vi "main.vi"() -> ()   [LabVIEW 2017]
uses:
  <vilib>/Instr/_visa.llb/VISA Set IO Buffer Mask.ctl
  <vilib>/Instr/_visa.llb/VISA Configure Serial Port (Instr).vi
panel:
  out "Pomiary":dynamicdata(graph)
  in  "stop":bool
  in  "VISA resource name":refnum<visa-resource-name>
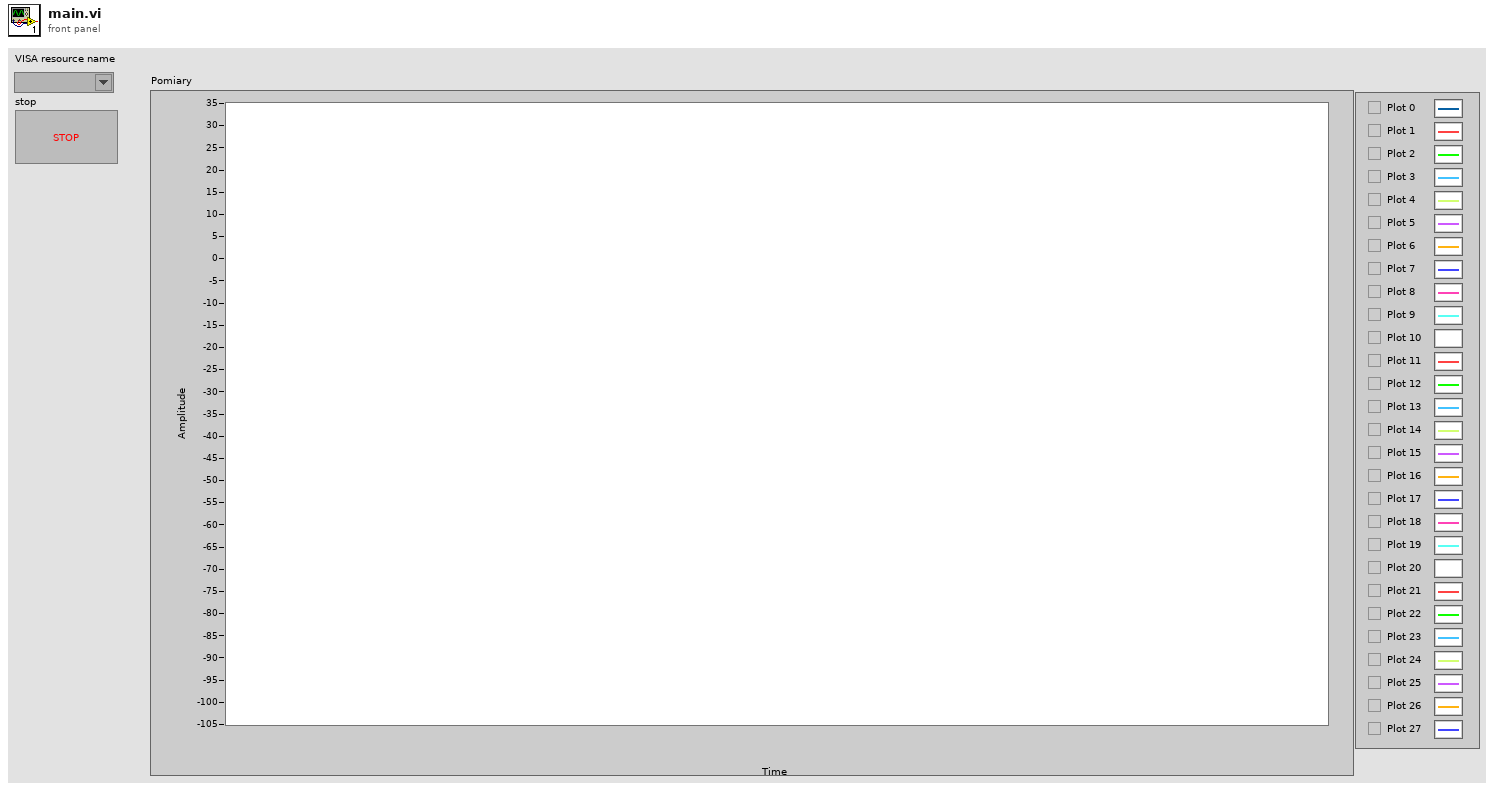
[diagram p1: front panel]
types:
  T1 = typedef "VISA Set IO Buffer Mask.ctl" = u16
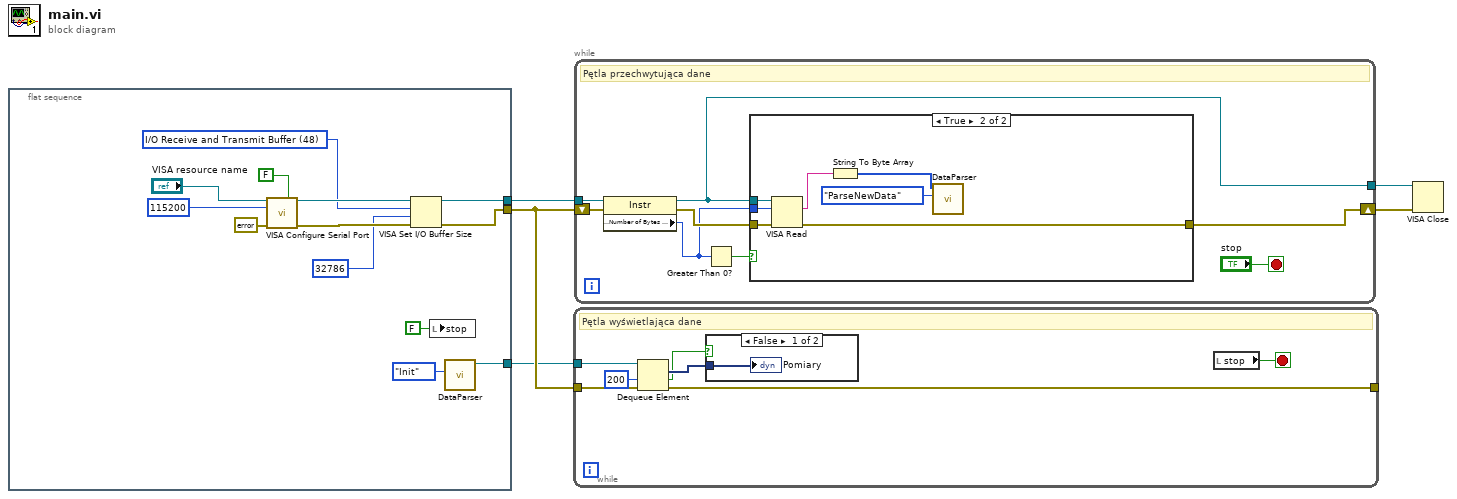
[diagram p0: block diagram]
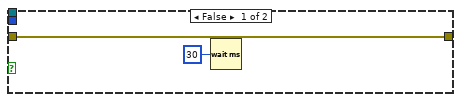
[diagram p3: hidden frame]
diagram:
  n1 = flat-sequence {
    tunnel: [w10] -> w4
    tunnel: [w12] -> w5
    tunnel: [w7] -> w3
    frame #0 {
      w9 = T1 48 items=["I/O Receive Buffer"=16, "I/O Transmit Buffer"=32, "I/O Receive and Transmit Buffer"=48] ("Mask")
      n2 = call-poly "VISA Configure Serial Port"("VISA resource name"="VISA resource name", "Enable Termination\nChar (T)"=FALSE ("Enable Termination\nChar (T)"), "baud rate (9600)"=u32 115200, "error in (no error)"=errorcluster {"status"=FALSE, "code"=0, "source"=""}) -> ("VISA resource name out"=w13:refnum<visa-resource-name>, "error out"=w11:errorcluster)  [unwired: 10 in]
      n3 = VISA Set I/O Buffer Size(VISA resource name=w13, mask (16)=w9, size (4096)=u32 32786, error in (no error)=w11) -> (VISA resource name out=w12:refnum<visa-resource-name>, error out=w10:errorcluster)
      n4 = local write "stop"(FALSE ("stop")) -> ()
      n5 = call "DataParser.vi"("Control"=enum16{"Init", "ParseNewData"}."Init") -> ("queue out"=w7:refnum<queue>)  [unwired: 10 in]
    }
  }
  n6 = while {
    tunnel: w4 -> [w24]
    tunnel: w3 -> [w25]
    tunnel: [w21] -> _
    stop <- w19 stop-if-true
    # "Pętla wyświetlająca dane"
    n7 = Dequeue Element(queue=w25, timeout in ms (-1)=200, error in (no error)=w24) -> (element=w22:dynamicdata, timed out?=w20:bool, error out=w21:errorcluster)  [unwired: 1 out]
    n8 = case shown="False" w20 {
      tunnel: w22 -> [w26 _]
      frame False {
        "Pomiary" <- w26
      }
      frame True {
      }
    }
    n9 = local read "stop"() -> (w19:bool)
  }
  n10 = while {
    tunnel: w5 -> [w33]
    shift-right: [w29] -> w2
    shift-left: w4 -> [w34]
    tunnel: [w27] -> w1
    stop <- "stop" stop-if-true
    # "Pętla przechwytująca dane"
    n11 = property class="Instr"(reference=w33, error in=w34) -> (reference out=w27:refnum<visa-resource-name>, error out=w32:errorcluster, "Serial Settings:Number of Bytes at Serial Port"=w31:u32)
    n12 = Greater Than 0?(x=w31) -> (x > 0?=w30:bool)
    n13 = case shown="True" w30 {
      tunnel: w27 -> [_ w43]
      tunnel: w32 -> [w35 w42]
      tunnel: w31 -> [_ w41]
      tunnel: [w35 w40] -> w29
      frame False {
        n14 = Wait (ms)(milliseconds to wait=u32 30) -> ()  [unwired: 1 out]
      }
      frame True {
        n15 = VISA Read(VISA resource name=w43, byte count=w41, error in (no error)=w42) -> (read buffer=w38:string, error out=w40:errorcluster)  [unwired: 2 out]
        n16 = String To Byte Array(string=w38) -> (unsigned byte array=w37:u8[])
        n17 = call "DataParser.vi"("Control"=enum16{"Init", "ParseNewData"}."ParseNewData", "NewData"=w37) -> ()  [unwired: 9 in, 1 out]
      }
    }
  }
  n18 = VISA Close(VISA resource name=w1, error in (no error)=w2) -> ()  [unwired: 1 out]
